vi "Error Display.vi"(11 "queue out":refnum<queue>) -> ()   [LabVIEW 2019, in "J1939 Workspace Shared.lvlib"]
uses:
  J1939 Workspace Shared.lvlib
  Addon/Addon Shared/Types/Error Cluster.ctl
  Addon/Addon Shared/Types/Error Types.ctl
  <vilib>/Utility/miscctls.llb/LVRowAndColumnUnsignedTypeDef.ctl
  Addon/Addon Shared/J1939 Addon Shared.lvlib
panel:
  in  "Clear":bool
  in  "Exit":bool
  in  "Error List":i32(listbox)
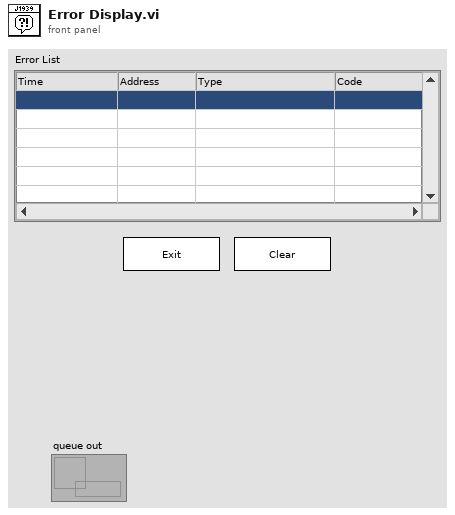
[diagram p1: front panel]
types:
  T1 = typedef "J1939 Addon Shared.lvlib/Error Cluster.ctl" = cluster{"error out":errorcluster, "Enum":T2, "Address":u8, "Timestamp":timestamp}
  T2 = typedef "J1939 Addon Shared.lvlib/Error Types.ctl" = enum16{"Request", "RAW Generation", "Clear Active DTCs", "Clear Previous DTCs", "Addresses", "TLAs", "Get Active DTCs", "Get Previous DTCs", "TCP Connection"}
  T3 = typedef "LVRowAndColumnUnsignedTypeDef.ctl" = cluster{"Row":u32, "Column":u32}
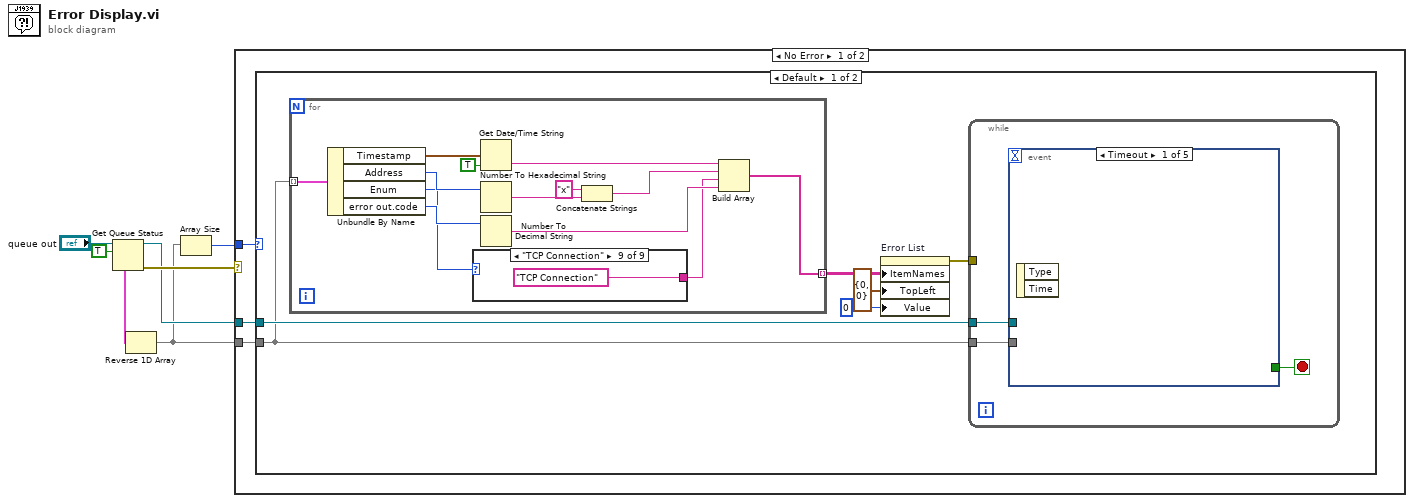
[diagram p0: block diagram]
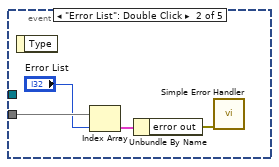
[diagram p2: hidden frame]
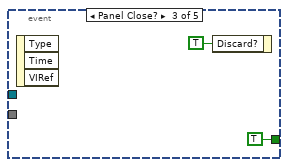
[diagram p3: hidden frame]
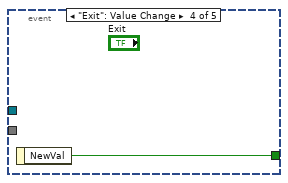
[diagram p4: hidden frame]
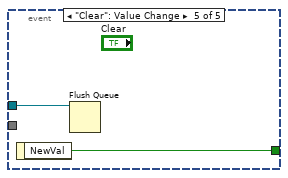
[diagram p5: hidden frame]
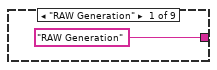
[diagram p6: hidden frame]
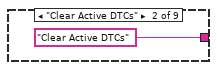
[diagram p7: hidden frame]
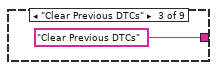
[diagram p8: hidden frame]
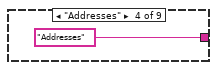
[diagram p9: hidden frame]
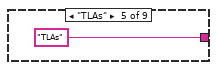
[diagram p10: hidden frame]
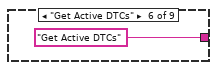
[diagram p11: hidden frame]
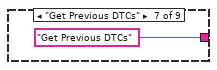
[diagram p12: hidden frame]
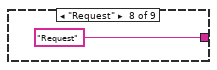
[diagram p13: hidden frame]
diagram:
  n1 = Get Queue Status(queue="queue out", return elements? (F)=TRUE) -> (queue out=w5:refnum<queue>, error out=w6:errorcluster, elements=w4:T1[])  [unwired: 1 in, 5 out]
  n2 = Reverse 1D Array(array=w4) -> (reversed array=w1:T1[])
  n3 = Array Size(array=w1) -> (size(s)=w3:i32)
  n4 = case shown="No Error" w6 {
    tunnel: w5 -> [w10 _]
    tunnel: w1 -> [w9 _]
    tunnel: w3 -> [w8 _]
    frame No Error {
      n5 = case shown="Default" w8 {
        tunnel: w10 -> [w14 _]
        tunnel: w9 -> [w13 _]
        frame Default {
          n6 = for {
            tunnel: w13 -> [w41] mode=indexing
            tunnel: [w35] -> w16 mode=indexing
            n7 = Unbundle By Name(w41) -> ("Timestamp"=w40:timestamp, "Address"=w37:u8, "Enum"=w32:T2, "error out.code"=w36:i32)
            n8 = case shown="\"TCP Connection\"" w32 {
              tunnel: ["RAW Generation" "Clear Active DTCs" "Clear Previous DTCs" "Addresses" "TLAs" "Get Active DTCs" "Get Previous DTCs" "Request" "TCP Connection"] -> w31
              frame "RAW Generation" {
              }
              frame "Clear Active DTCs" {
              }
              frame "Clear Previous DTCs" {
              }
              frame "Addresses" {
              }
              frame "TLAs" {
              }
              frame "Get Active DTCs" {
              }
              frame "Get Previous DTCs" {
              }
              frame "Request" {
              }
              frame "TCP Connection" {
              }
            }
            n9 = Get Date/Time String(seconds (now)=w40, want seconds? (F)=TRUE) -> (time string=w38:string)  [unwired: 1 in, 1 out]
            n10 = Number To Hexadecimal String(2:w37) -> (0:w34:string)  [unwired: 1 in]
            n11 = Number To Decimal String(number=w36) -> (decimal integer string=w33:string)  [unwired: 1 in]
            n12 = Concatenate Strings("x" ("string"), w34) -> (w30:string)
            n13 = Build Array(w38, w30, w31, w33) -> (w35:string[])
          }
          n14 = property on="Error List" class="MCListbox (strict)"("ItemNames"=w16, "TopLeft"=T3 {"Row"=0, "Column"=0} ("Top Left Visible Cell"), "Value"=0 ("Error List")) -> (error out=w15:errorcluster)  [unwired: 2 in, 1 out]
          n15 = while {
            tunnel: w15 -> [_]
            tunnel: w13 -> [w19]
            tunnel: w14 -> [w17]
            stop <- w18 stop-if-true
            n16 = event shown="[0] Timeout" {
              selector: _ -> [_ _ _ _ _]
              dyn-events: _ -> [_ _ _ _ _]
              timeout: _ -> [_ _ _ _ _]
              tunnel: w19 -> [_ w23 _ _ _]
              tunnel: [_ _ TRUE ("NewVal") w26 w28] -> w18
              tunnel: w17 -> [_ _ _ _ w27]
              event Timeout {
                n17 = event-data() -> ()  [unwired: 1 in, 2 out]
              }
              event "Error List": Double Click {
                n18 = event-data() -> ()  [unwired: 1 in, 1 out]
                n19 = Index Array(array=w23, index="Error List") -> (element=w21:T1)
                n20 = Unbundle By Name(w21) -> ("error out"=w20:errorcluster)
                n21 = call <vilib>:"Simple Error Handler.vi"("error in (no error)"=w20) -> ()  [unwired: 4 in, 5 out]
              }
              event Panel Close? {
                n22 = event-data() -> ()  [unwired: 1 in, 3 out]
                n23 = event-data("Discard?"=TRUE) -> ()  [unwired: 1 in, 1 out]
              }
              event "Exit": Value Change {
                n24 = event-data() -> ("NewVal"=w26:bool)  [unwired: 1 in]
              }
              event "Clear": Value Change {
                n25 = event-data() -> ("NewVal"=w28:bool)  [unwired: 1 in]
                n26 = Flush Queue(queue=w27) -> ()  [unwired: 1 in, 3 out]
              }
            }
          }
        }
        frame 0 {
        }
      }
    }
    frame Error {
    }
  }
